vi "Execute.UI.Complete.vi"(8 "error in (no error)":errorcluster, 11 "Cluster":T1) -> (0 "error out":errorcluster)   [LabVIEW 2013, in "Simple Sequence Editor.lvlib"]
uses:
  Simple Sequence Editor.lvlib
  Types/Execuction.StateVariables.ctl
  <vilib>/NI Veristand/Execution/Workspace/SystemStateRegEventRef.ctl
  <vilib>/NI Veristand/Execution/Workspace/SystemStateEventRef.ctl
  <vilib>/NI Veristand/Execution/Workspace/WorkspaceAPI.ctl
  NationalInstruments.VeriStand.ClientAPI
  NationalInstruments.VeriStand.RealTimeSequenceDefinitionApi
  Program Files/National Instruments/LabVIEW 2013/examples/NI Veristand/API/Execution API/Sequences/Stimulus Profile Control Tool/Project Execution State.ctl
  <vilib>/NI Veristand/Execution/Workspace/NI_VS Workspace ExecutionAPI.lvlib
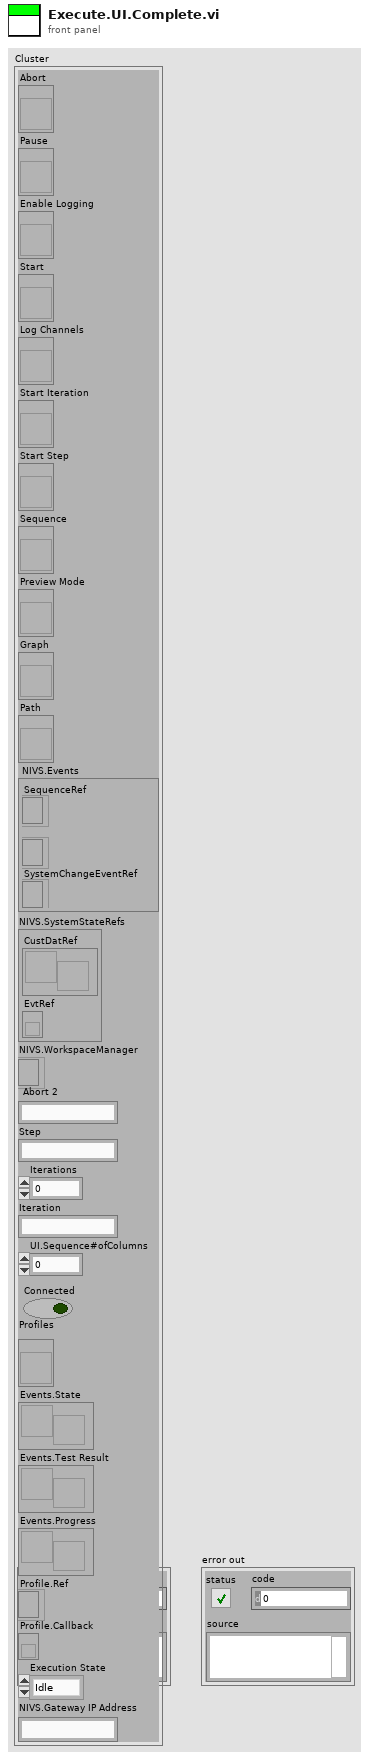
[diagram p1: front panel]
types:
  T1 = typedef "Simple Sequence Editor.lvlib/Execuction.StateVariables.ctl" = cluster{"Abort":refnum<vi>, "Pause":refnum<vi>, "Enable Logging":refnum<vi>, "Start":refnum<vi>, "Log Channels":refnum<vi>, "Start Iteration":refnum<vi>, "Start Step":refnum<vi>, "Sequence":refnum<vi>, "Preview Mode":refnum<vi>, "Graph":refnum<vi>, "Path":refnum<vi>, "NIVS.Events":cluster{"SequenceRef":refnum<event-registration>, "NIVS.Workspace Event":refnum<event-registration>, "SystemChangeEventRef":T2}, "NIVS.SystemStateRefs":T3, "NIVS.WorkspaceManager":T4, "Abort 2":string, "Step":string, "Iterations":u32, "Iteration":string, "UI.Sequence#ofColumns":i32, "Connected":bool, "Profiles":refnum<vi>, "Events.State":refnum<user-event>, "Events.Test Result":refnum<user-event>, "Events.Progress":refnum<user-event>, "Profile.Ref":refnum<k24>, "Profile.Callback":refnum<k27>, "State":T5, "NIVS.Gateway IP Address":string}
  T2 = typedef "NI_VS Workspace ExecutionAPI.lvlib/SystemStateRegEventRef.ctl" = refnum<event-registration>
  T3 = typedef "NI_VS Workspace ExecutionAPI.lvlib/SystemStateEventRef.ctl" = cluster{"CustDatRef":refnum<user-event>, "EvtRef":refnum<k27>}
  T4 = typedef "NI_VS Workspace ExecutionAPI.lvlib/WorkspaceAPI.ctl" = refnum<k24>
  T5 = typedef "Project Execution State.ctl" = enum16{"Idle", "Initializing", "Running", "Paused", "Finalizing", "Complete"}
  T6 = enum8{"Enabled", "Disabled", "Disabled and Grayed Out"}
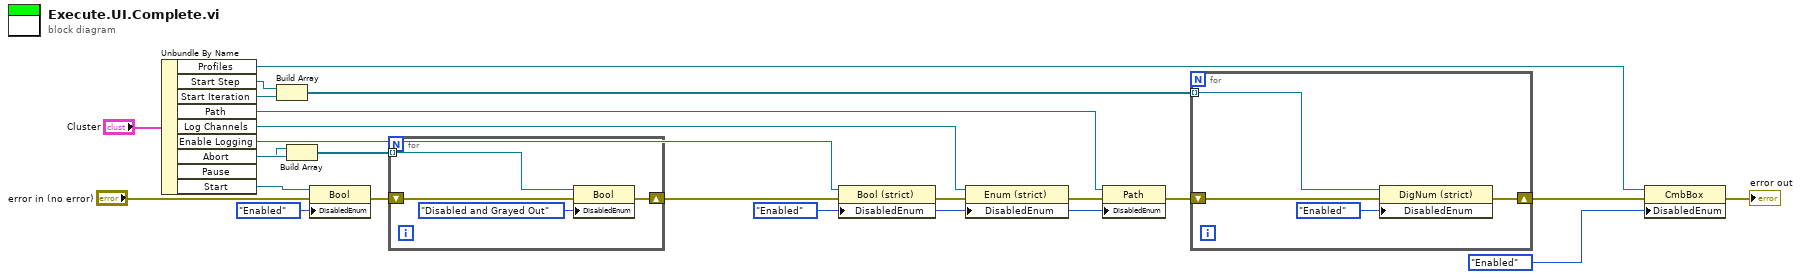
[diagram p0: block diagram]
diagram:
  w5 = T6."Enabled" ("Disabled")
  n1 = Unbundle By Name("Cluster") -> ("Profiles"=w23:refnum<vi>, "Start Step"=w20:refnum<vi>, "Start Iteration"=w19:refnum<vi>, "Path"=w6:refnum<vi>, "Log Channels"=w17:refnum<vi>, "Enable Logging"=w16:refnum<vi>, "Abort"=w12:refnum<vi>, "Pause"=w13:refnum<vi>, "Start"=w7:refnum<vi>)
  n2 = Build Array(w20, w19) -> (w21:refnum<vi>[])
  n3 = Build Array(w12, w13) -> (w14:refnum<vi>[])
  n4 = property class="Bool"(reference=w7, error in="error in (no error)", "DisabledEnum"=T6."Enabled" ("Disabled")) -> (error out=w8:errorcluster)  [unwired: 1 out]
  n5 = for {
    tunnel: w14 -> [w27] mode=indexing
    shift-right: [w25] -> w15
    shift-left: w8 -> [w24]
    n6 = property class="Bool"(reference=w27, error in=w24, "DisabledEnum"=T6."Disabled and Grayed Out" ("Disabled")) -> (error out=w25:errorcluster)  [unwired: 1 out]
  }
  n7 = property class="Bool (strict)"(reference=w16, error in=w15, "DisabledEnum"=w5) -> (error out=w18:errorcluster)  [unwired: 1 out]
  n8 = property class="Enum (strict)"(reference=w17, error in=w18, "DisabledEnum"=w5) -> (error out=w4:errorcluster)  [unwired: 1 out]
  n9 = property class="Path"(reference=w6, error in=w4, "DisabledEnum"=w5) -> (error out=w3:errorcluster)  [unwired: 1 out]
  n10 = for {
    tunnel: w21 -> [w31] mode=indexing
    shift-right: [w29] -> w22
    shift-left: w3 -> [w28]
    n11 = property class="DigNum (strict)"(reference=w31, error in=w28, "DisabledEnum"=T6."Enabled" ("Disabled")) -> (error out=w29:errorcluster)  [unwired: 1 out]
  }
  n12 = property class="CmbBox"(reference=w23, error in=w22, "DisabledEnum"=T6."Enabled" ("Disabled")) -> (error out=→"error out":errorcluster)  [unwired: 1 out]
